vi "ContFindFit.vi"(8 "error in (no error)":errorcluster, 9 "GenImage":bool, 10 "update":bool, 11 "Compiler Settings":T1={"Python Path"=path "", "Main File"="mainscript.py", "Meta File"="metascript.txt", "Aux File"="auxscript.py", "Pre File"="metascript.txt"}) -> (0 "error out":errorcluster)   [LabVIEW 2019]
uses:
  PulseCompiler/CompilerSettings.ctl
  controls/GlobalExp.vi
  Log/GlobalPyConsole.vi
  Global.lvlib
panel:
  out "standard output":string
  out "standard error":string
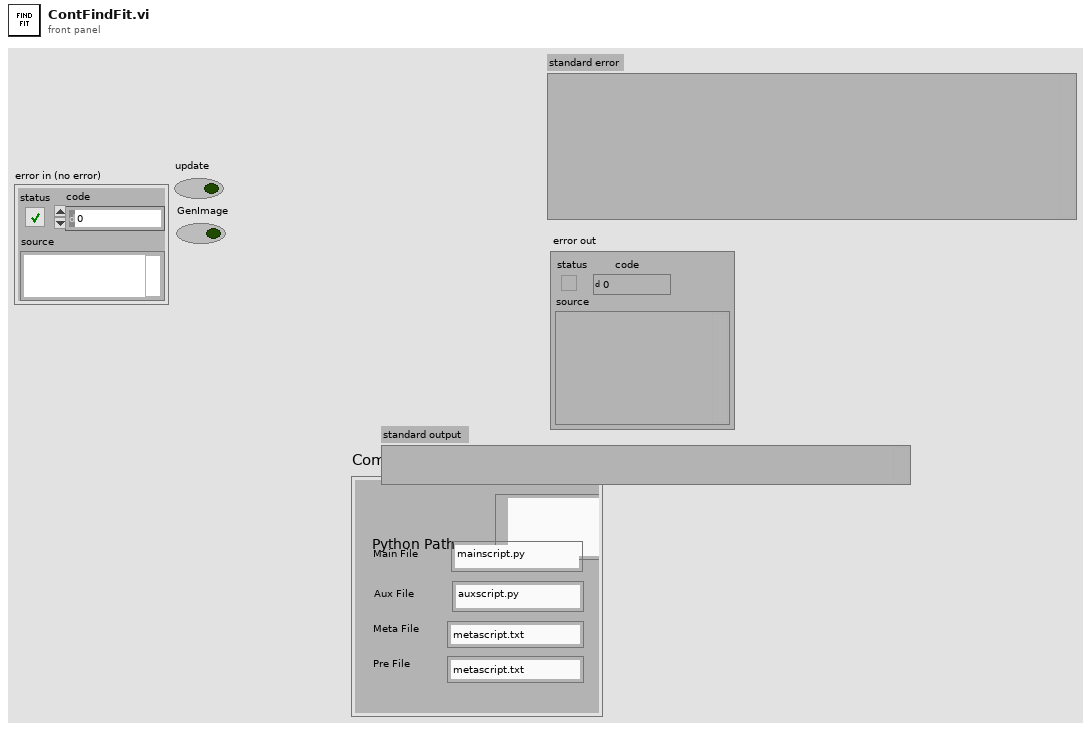
[diagram p1: front panel]
types:
  T1 = typedef "CompilerSettings.ctl" = cluster{"Python Path":path, "Main File":string, "Meta File":string, "Aux File":string, "Pre File":string}
  T2 = cluster{"date":string, "expnum":string, "update":bool, "genimage":bool}
  T3 = typedef "MasterExpControl.ctl" = cluster{"Main Steps":dbl, "Main Runs":dbl, "ExpStatus":enum16{"Innit", "Stop", "Idle", "MainRunning", "AuxRunning"}, "Main Current Step":dbl, "ExpNum":dbl, "NewData":bool, "date":string, "command":string, "Stop":bool, "Pause":bool, "Mathematica":string, "Main/Meta":bool, "UpdateMath":bool, "Camera":bool, "MetaExpOver":bool, "NextMetaExp":bool}
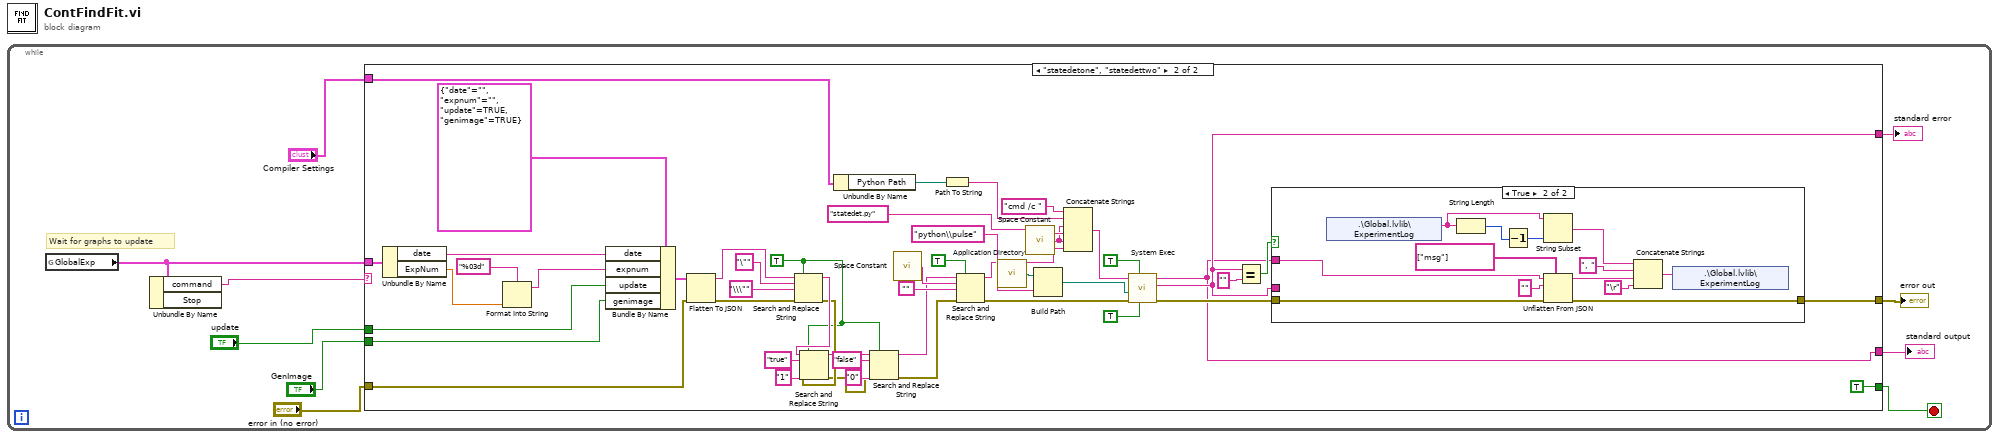
[diagram p0: block diagram]
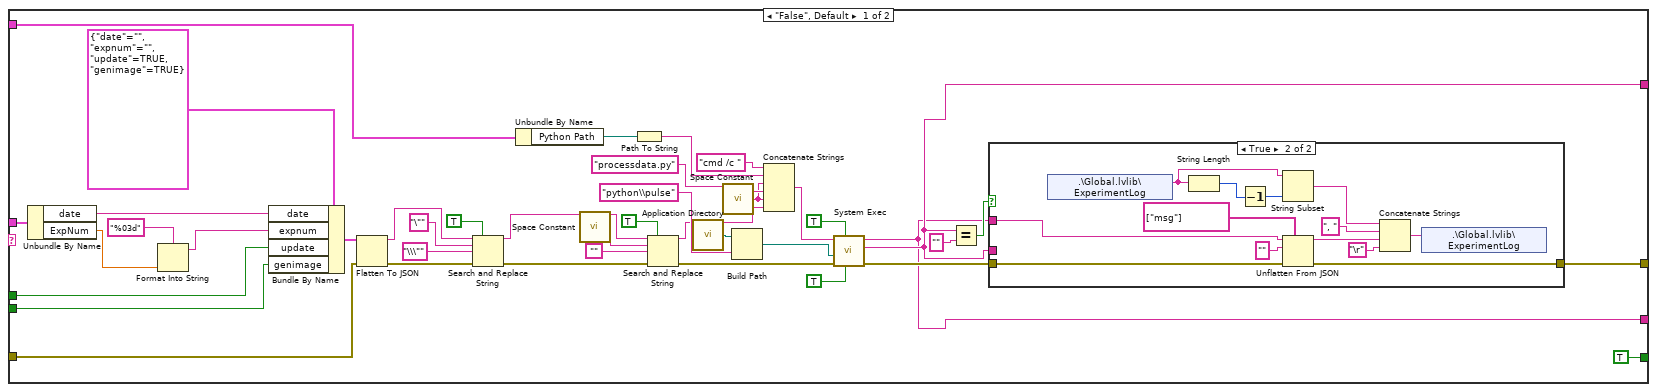
[diagram p2: hidden frame]
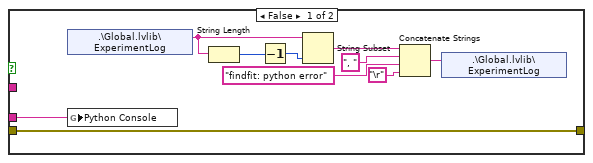
[diagram p3: hidden frame]
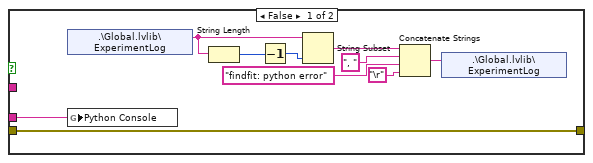
[diagram p4: hidden frame]
diagram:
  n1 = while {
    stop <- w2 stop-if-true
    # "Wait for graphs to update"
    n2 = global read "GlobalExp.vi" "GlobalExp"() -> (w10:T3)
    n3 = Unbundle By Name(w10) -> ("command"=w9:string)  [unwired: 1 out]
    n4 = case shown="\"statedetone\", \"statedettwo\"" w9 {
      tunnel: w10 -> [w24 w99]
      tunnel: [TRUE TRUE] -> w2
      tunnel: "update" -> [w17 w92]
      tunnel: "GenImage" -> [w16 w91]
      tunnel: [w15 w87] -> w6
      tunnel: [w14 w89] -> w5
      tunnel: [w13 w88] -> w4
      tunnel: "error in (no error)" -> [w12 w90]
      tunnel: "Compiler Settings" -> [w11 w86]
      frame "False", Default {
        n5 = Unbundle By Name(w24) -> ("date"=w28:string, "ExpNum"=w26:dbl)
        n6 = Format Into String(format string="%03d", w26) -> (resulting string=w27:string)  [unwired: 2 in, 1 out]
        n7 = Bundle By Name(cluster=T2 {"date"="", "expnum"="", "update"=TRUE, "genimage"=TRUE}, "date"=w28, "expnum"=w27, "update"=w17, "genimage"=w16) -> (w29:T2)
        n8 = Flatten To JSON(anything=w29, error in (no error)=w12) -> (JSON string=w42:string, 11:w41:errorcluster)  [unwired: 1 in]
        n9 = Search and Replace String(replace all?=TRUE ("replace all? (F)"), input string=w42, search string="\"", replace string="\\\"" ("replace string (\"\")"), error in=w41) -> (result string=w38:string, error out=w37:errorcluster)  [unwired: 3 in, 2 out]
        n10 = Unbundle By Name(w11) -> ("Python Path"=w21:path)
        n11 = call <vilib>:"Space Constant.vi"() -> ("String"=w36:string)
        n12 = Path To String(path=w21) -> (string=w20:string)
        n13 = Search and Replace String(replace all?=TRUE ("replace all? (F)"), input string=w38, search string=w36, replace string="", error in=w37) -> (result string=w34:string, error out=w33:errorcluster)  [unwired: 3 in, 2 out]
        n14 = call <vilib>:"Application Directory.vi"() -> ("Application Directory"=w46:path)
        n15 = call <vilib>:"Space Constant.vi"() -> ("String"=w43:string)
        n16 = Build Path(base path=w46, name or relative path="python\\pulse") -> (appended path=w48:path)
        n17 = Concatenate Strings("cmd /c " ("string"), w20, w43, "processdata.py" ("name or relative path"), w43, w34) -> (w45:string)
        n18 = call <vilib>:"System Exec.vi"("run minimized? (F)"=TRUE, "wait until completion? (T)"=TRUE, "error in (no error)"=w33, "working directory"=w48, "command line"=w45) -> ("error out"=w22:errorcluster, "standard error"=w14:string, "standard output"=w13:string)  [unwired: 3 in, 1 out]
        n19 = Equal?(x=w14, y="") -> (x = y?=w18:bool)
        n20 = case shown="True" w18 {
          tunnel: w13 -> [_ w73]
          tunnel: w22 -> [w61 w70]
          tunnel: [w61 w62] -> w15
          tunnel: w14 -> [w60 _]
          frame False {
            n21 = shared-variable ".\\Global.lvlib\\ExperimentLog"() -> (w53:string)  [unwired: 1 in, 1 out]
            n22 = global write "GlobalPyConsole.vi" "Python Console"(w60) -> ()
            n23 = String Length(string=w53) -> (length=w57:i32)
            n24 = Decrement(x=w57) -> (x-1=w58:i32)
            n25 = String Subset(string=w53, length (rest)=w58) -> (substring=w56:string)  [unwired: 1 in]
            n26 = Concatenate Strings(w56, ", " ("string"), "findfit: python error" ("string"), "\r") -> (w59:string)
            n27 = shared-variable ".\\Global.lvlib\\ExperimentLog"(w59) -> ()  [unwired: 1 in, 1 out]
          }
          frame True {
            n28 = shared-variable ".\\Global.lvlib\\ExperimentLog"() -> (w69:string)  [unwired: 1 in, 1 out]
            n29 = String Length(string=w69) -> (length=w67:i32)
            n30 = Decrement(x=w67) -> (x-1=w68:i32)
            n31 = String Subset(string=w69, length (rest)=w68) -> (substring=w65:string)  [unwired: 1 in]
            n32 = Unflatten From JSON(path=string[] ["msg"], JSON string=w73, type and defaults="", error in (no error)=w70) -> (value=w66:string, error out=w62:errorcluster)  [unwired: 3 in]
            n33 = Concatenate Strings(w65, ", " ("string"), w66, "\r") -> (w74:string)
            n34 = shared-variable ".\\Global.lvlib\\ExperimentLog"(w74) -> ()  [unwired: 1 in, 1 out]
          }
        }
      }
      frame "statedetone", "statedettwo" {
        w80 = TRUE ("replace all? (F)")
        n35 = Unbundle By Name(w99) -> ("date"=w103:string, "ExpNum"=w101:dbl)
        n36 = Format Into String(format string="%03d", w101) -> (resulting string=w102:string)  [unwired: 2 in, 1 out]
        n37 = Bundle By Name(cluster=T2 {"date"="", "expnum"="", "update"=TRUE, "genimage"=TRUE}, "date"=w103, "expnum"=w102, "update"=w92, "genimage"=w91) -> (w104:T2)
        n38 = Flatten To JSON(anything=w104, error in (no error)=w90) -> (JSON string=w114:string, 11:w113:errorcluster)  [unwired: 1 in]
        n39 = Search and Replace String(replace all?=w80, input string=w114, search string="\"", replace string="\\\"" ("replace string (\"\")"), error in=w113) -> (result string=w85:string, error out=w82:errorcluster)  [unwired: 3 in, 2 out]
        n40 = Search and Replace String(replace all?=w80, input string=w85, search string="true", replace string="1" ("replace string (\"\")"), error in=w82) -> (result string=w81:string, error out=w77:errorcluster)  [unwired: 3 in, 2 out]
        n41 = Unbundle By Name(w86) -> ("Python Path"=w96:path)
        n42 = Search and Replace String(replace all?=w80, input string=w81, search string="false", replace string="0" ("replace string (\"\")"), error in=w77) -> (result string=w75:string, error out=w76:errorcluster)  [unwired: 3 in, 2 out]
        n43 = call <vilib>:"Space Constant.vi"() -> ("String"=w110:string)
        n44 = Path To String(path=w96) -> (string=w95:string)
        n45 = Search and Replace String(replace all?=TRUE ("replace all? (F)"), input string=w75, search string=w110, replace string="", error in=w76) -> (result string=w108:string, error out=w107:errorcluster)  [unwired: 3 in, 2 out]
        n46 = call <vilib>:"Application Directory.vi"() -> ("Application Directory"=w118:path)
        n47 = call <vilib>:"Space Constant.vi"() -> ("String"=w115:string)
        n48 = Build Path(base path=w118, name or relative path="python\\pulse") -> (appended path=w120:path)
        n49 = Concatenate Strings("cmd /c " ("string"), w95, w115, "statedet.py" ("name or relative path"), w115, w108) -> (w117:string)
        n50 = call <vilib>:"System Exec.vi"("run minimized? (F)"=TRUE, "wait until completion? (T)"=TRUE, "error in (no error)"=w107, "working directory"=w120, "command line"=w117) -> ("error out"=w97:errorcluster, "standard error"=w89:string, "standard output"=w88:string)  [unwired: 3 in, 1 out]
        n51 = Equal?(x=w89, y="") -> (x = y?=w93:bool)
        n52 = case shown="True" w93 {
          tunnel: w88 -> [_ w145]
          tunnel: w97 -> [w133 w142]
          tunnel: [w133 w134] -> w87
          tunnel: w89 -> [w132 _]
          frame False {
            n53 = shared-variable ".\\Global.lvlib\\ExperimentLog"() -> (w125:string)  [unwired: 1 in, 1 out]
            n54 = global write "GlobalPyConsole.vi" "Python Console"(w132) -> ()
            n55 = String Length(string=w125) -> (length=w129:i32)
            n56 = Decrement(x=w129) -> (x-1=w130:i32)
            n57 = String Subset(string=w125, length (rest)=w130) -> (substring=w128:string)  [unwired: 1 in]
            n58 = Concatenate Strings(w128, ", " ("string"), "findfit: python error" ("string"), "\r") -> (w131:string)
            n59 = shared-variable ".\\Global.lvlib\\ExperimentLog"(w131) -> ()  [unwired: 1 in, 1 out]
          }
          frame True {
            n60 = shared-variable ".\\Global.lvlib\\ExperimentLog"() -> (w141:string)  [unwired: 1 in, 1 out]
            n61 = String Length(string=w141) -> (length=w139:i32)
            n62 = Decrement(x=w139) -> (x-1=w140:i32)
            n63 = String Subset(string=w141, length (rest)=w140) -> (substring=w137:string)  [unwired: 1 in]
            n64 = Unflatten From JSON(path=string[] ["msg"], JSON string=w145, type and defaults="", error in (no error)=w142) -> (value=w138:string, error out=w134:errorcluster)  [unwired: 3 in]
            n65 = Concatenate Strings(w137, ", " ("string"), w138, "\r") -> (w146:string)
            n66 = shared-variable ".\\Global.lvlib\\ExperimentLog"(w146) -> ()  [unwired: 1 in, 1 out]
          }
        }
      }
    }
    "error out" <- w6
    "standard error" <- w5
    "standard output" <- w4
  }
